vi "Dashboard Main.vi"() -> ()   [LabVIEW 2019]
uses:
  <vilib>/Rock Robotics/Network Tables/NT Read Numeric Array.vi
  <vilib>/Rock Robotics/Network Tables/NT Read String.vi
  max2018/dashboard/src/Robot Starting Location.ctl
panel:
  out "Camera Perf":string
  in  "Camera Settings":T1={"Frame Rate"=30, "Compression"=30, "Size"=1, "DB Camera Config"=FALSE} {"Frame Rate" scale=1.0..30.0; "Compression" scale=100.0..-1.0; "Size" items=["640x480", "320x240", "160x120"]}
  in  "TCP":refnum<k5>
  out "Robot IP":string
  in  "Dashboard Tab":enum32{"Drive", "Basic", "Custom", "Variables"}(tab)
  out "String":string
  in  "Robot Starting Location":enum32{"Left", "Centre", "Right", "Straight"}(radio)=enum."Centre"
  out "NT Connection":bool
  out "MotorChart R":cluster{"Numeric":dbl, "Numeric":dbl}(graph)
  out "MotorChart L":cluster{"Numeric":dbl, "Numeric":dbl}(graph)
  out "MotorSliders R":cluster{"MotorSlide1":dbl, "MotorSlide2":dbl} {"MotorSlide2" scale=-1.0..1.0 scale format="%#_2e"; "MotorSlide1" scale=-1.0..1.0 scale format="%#_2e"}
  out "MotorSliders L":cluster{"MotorSlide1":dbl, "MotorSlide2":dbl} {"MotorSlide2" scale=-1.0..1.0 scale format="%#_2e"; "MotorSlide1" scale=-1.0..1.0 scale format="%#_2e"}
  out "JS1 Z":dbl(slide) scale=-1.0..1.0 scale format="%#_2e"
  out "JS1 Graph":cluster{"X":dbl, "Y":dbl}[](graph)
  out "JS1 Buttons":T2
  out "JS2 Z":dbl(slide) scale=-1.0..1.0 scale format="%#_2e"
  out "JS2 Graph":cluster{"X":dbl, "Y":dbl}[](graph)
  out "JS2 Buttons":T2
  out "Mode":T3(ring)=enum."Auto Disabled"
  in  "DB/String 9":string
  in  "DB/String 8":string
  in  "DB/String 7":string
  in  "DB/String 6":string
  in  "DB/String 5":string
  in  "DB/String 4":string
  in  "DB/String 3":string
  in  "DB/String 2":string
  in  "DB/String 1":string
  in  "DB/String 0":string
  in  "DB/Slider 0":dbl(slide) scale=0.0..5.0
  in  "DB/Slider 1":dbl(slide) scale=0.0..5.0
  in  "DB/Slider 2":dbl(slide) scale=0.0..5.0
  in  "DB/Slider 3":dbl(slide) scale=0.0..5.0
  out "DB/LED 3":bool
  out "DB/LED 2":bool
  out "DB/LED 1":bool
  out "DB/LED 0":bool
  in  "DB/Button 3":bool
  in  "DB/Button 2":bool
  in  "DB/Button 1":bool
  in  "DB/Button 0":bool caption="New Name"
  out "Tree":string(tree)
  out "Camera Image":T4(plugin-control)
  in  "Camera Name":string(combo)="No Camera Selection"
  # "HW"
  # "Joysticks"
  # "Drive Motors"
  # "Front"
  # "Right"
  # "Left"
  # "Back"
  # "This tab is a great place for autonomous settings and robot-specific values.\nPlace controls and indicators inside this tab and match name to\nDashboard Variables on robot. You can also delete this comment."
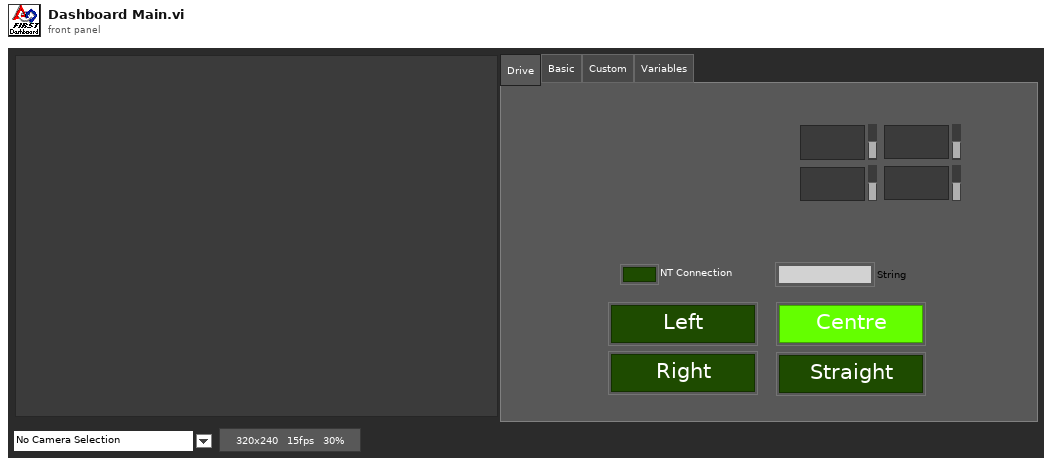
[diagram p1: front panel]
types:
  T1 = cluster{"Frame Rate":i32, "Compression":i32, "Size":u16, "DB Camera Config":bool}
  T2 = cluster{bool, bool, bool, bool, bool, bool, bool, bool, bool, bool, bool, bool}
  T3 = enum8{"Tele-Op Disabled", "Tele-Op Enabled", "Auto Disabled", "Auto Enabled", "Test Disabled", "Test Enabled", "Disconnected", "No Code", "E-Stop"}
  T4 = typedef "IMAQ Image.ctl" = refnum<image>
  T5 = typedef "Robot Starting Location.ctl" = enum32{"Left", "Centre", "Right"}
  T6 = cluster{"Save Path":path, "Interval (s)":dbl, "Keep":i32}
  T7 = typedef "Image Type" = u32
  T8 = cluster{"Camera Image":refnum<vi>, "Dashboard Tab":refnum<vi>, void, "Tree":refnum<vi>, "Camera Settings":refnum<vi>, "Camera Name":refnum<vi>, "Camera Perf":refnum<vi>}
  T9 = cluster{"Shift":bool, "Ctrl":bool, "Alt":bool, "Cmd":bool, "Opt":bool}
  T10 = cluster{"Error Strings":string, "Disable Counts":cluster{u16, u16}, "Rail Faults":cluster{u16, u16, u16}, "Robot IP":string, "DB Mode":u8, "Event Info":cluster{"Name":string, "Type":u8, "Number":u16, "Replay":u8}}
  T11 = cluster{"Storage":cluster{"Disk Free":u64, "RAM Block":u32, "RAM free":u32}, "CPU Utilization":cluster{"CPU % ISR":sgl, "CPU % Time Crit":sgl, "CPU % Timed Str":sgl, "CPU % High":sgl, "CPU % Above":sgl, "CPU % Normal":sgl, "CPU % Low":sgl}, "CAN":cluster{"% Bus Utilization":sgl, "Bus Off Cnt":u32, "TX_FIFO Full Cnt":u32, "Receive Error Cnt":u8, "Transmit Error Cnt":u8}, "HID":cluster{"HID Outputs":u32, "Rumble Low":u16, "Rumble High":u16}[]}
  T12 = cluster{"Status bits":cluster{"Test Mode":bool, "Autonomous":bool, "Enabled":bool, "Code Start":bool, "Brownout":bool, "Reserved 2":bool, "Reserved 3":bool, "E-Stop":bool}, "Code Trace":cluster{"Disabled":bool, "TeleOp":bool, "Auto":bool, "Test":bool}, "Controller Type":enum16{"unknown", "cRIO", "roboRio"}, "Code?":enum16{"unknown", "noCode", "code"}, "Battery V":dbl}
  T13 = cluster{"Control Bits":cluster{"TestMode":bool, "Autonomous":bool, "Enabled":bool, "FMS Present":bool, bool, bool, bool, "E-Stop":bool}, "Team Station ":u8, "Countdown":sgl, "Joystick Values":cluster{"Axes":dbl[], "Buttons":bool[], "POVs":i16[]}[]}
  T14 = cluster{"Axes":dbl[], "Buttons":bool[], "POVs":i16[]}[]
  T15 = cluster{"Axes":dbl[], "Buttons":bool[], "POVs":i16[]}
  T16 = cluster{"Buttons[0]":bool, "Buttons[1]":bool, "Buttons[2]":bool, "Buttons[3]":bool, "Buttons[4]":bool, "Buttons[5]":bool, "Buttons[6]":bool, "Buttons[7]":bool, "Buttons[8]":bool, "Buttons[9]":bool, "Buttons[10]":bool, "Buttons[11]":bool}
  T17 = cluster{"Camera Name":string, "Camera File Name":string, "Saved DB Images Info":cluster{"Save Path":path, "Interval (s)":dbl, "Keep":i32}}
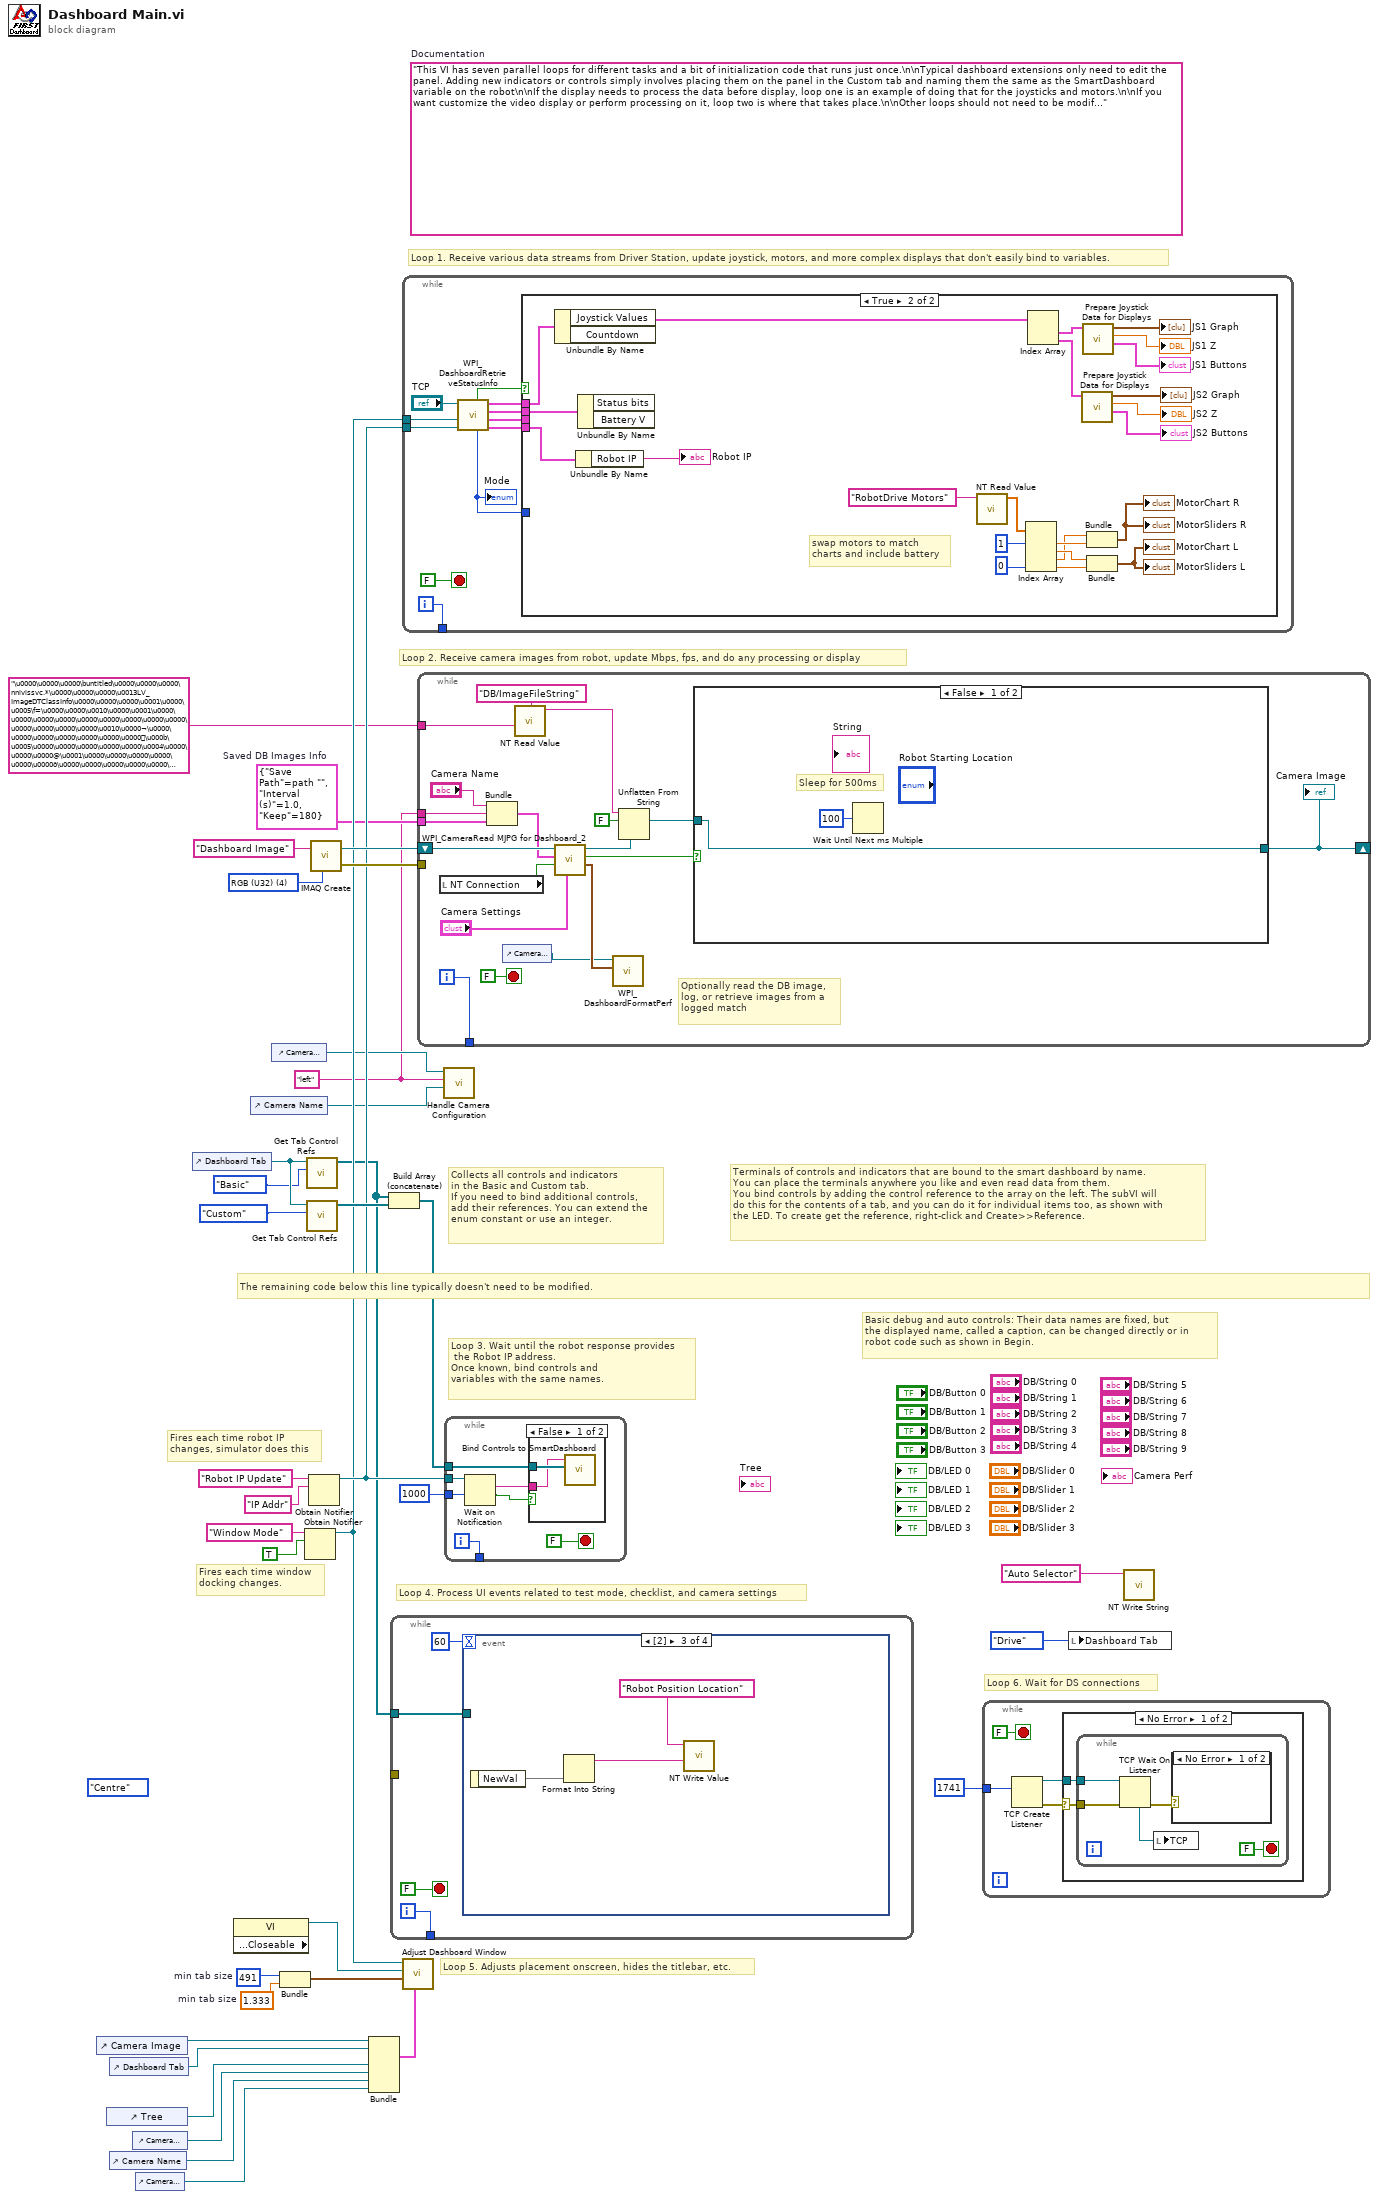
[diagram p0: block diagram]
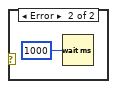
[diagram p2: hidden frame]
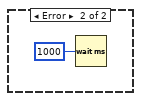
[diagram p3: hidden frame]
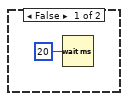
[diagram p4: hidden frame]
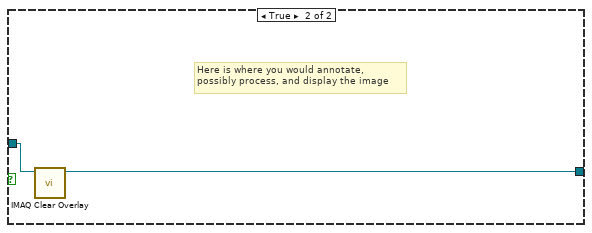
[diagram p6: hidden frame]
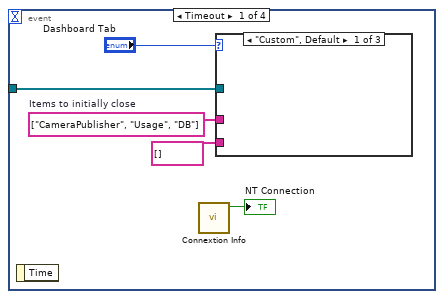
[diagram p7: hidden frame]
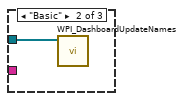
[diagram p8: hidden frame]
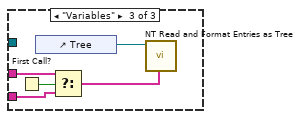
[diagram p9: hidden frame]
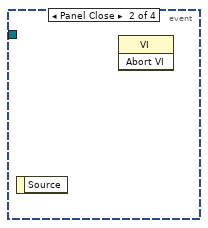
[diagram p10: hidden frame]
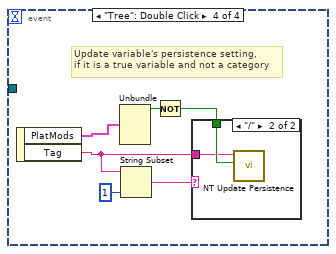
[diagram p11: hidden frame]
diagram:
  w2 = Robot_Starting_Location."Centre" ("Value (Signaling)")
  w4 = "left" ("Camera File Name")
  w5 = T6 {"Save Path"=path "", "Interval (s)"=1.0, "Keep"=180}  # Saved DB Images Info
  w25 = 491  # min tab size
  w24 = 1.333  # min tab size
  (unwired) "This VI has seven parallel loops for different tasks and a bit of initialization code that runs just once.\n\nTypical dashboard extensions only need to edit the panel. Adding new indicators or controls simply involves placing them on the panel in the Custom tab and naming them the same as the SmartDashboard variable on the robot\n\nIf the display needs to process the data before display, loop one is an example of doing that for the joysticks and motors.\n\nIf you want customize the video display or perform processing on it, loop two is where that takes place.\n\nOther loops should not need to be modified. They are pretty standard, and document the task they perform."  # Documentation
  w40 = T7 4 items=["Grayscale (U8)", "Grayscale (I16)", "Grayscale (SGL)", "Complex (CSG)", "RGB (U32)", "HSL (U32)", "RGB (U64)"] ("Image Type")
  # "Loop 6. Wait for DS connections"
  # "Basic debug and auto controls: Their data names are fixed, but\nthe displayed name, called a caption, can be changed directly or in\nrobot code such as shown in Begin."
  # "Fires each time robot IP\nchanges, simulator does this"
  # "Fires each time window\ndocking changes."
  # "Collects all controls and indicators\nin the Basic and Custom tab.\nIf you need to bind additional controls,\nadd their references. You can extend the\nenum constant or use an integer."
  # "The remaining code below this line typically doesn't need to be modified."
  # "Loop 4. Process UI events related to test mode, checklist, and camera settings"
  # "Terminals of controls and indicators that are bound to the smart dashboard by name.\nYou can place the terminals anywhere you like and even read data from them.\nYou bind controls by adding the control reference to the array on the left. The subVI will\ndo this for the contents of a tab, and you can do it for individual items too, as shown with\nthe LED. To create get the reference, right-click and Create>>Reference."
  # "Loop 3. Wait until the robot response provides\n the Robot IP address.\nOnce known, bind controls and\nvariables with the same names."
  # "Loop 5. Adjusts placement onscreen, hides the titlebar, etc."
  # "Loop 1. Receive various data streams from Driver Station, update joystick, motors, and more complex displays that don't easily bind to variables."
  # "Loop 2. Receive camera images from robot, update Mbps, fps, and do any processing or display"
  n1 = control-ref of="Camera Image"() -> (w27:refnum<vi>)
  n2 = control-ref of="Tree"() -> (w11:refnum<vi>)
  n3 = control-ref of="Dashboard Tab"() -> (w26:refnum<vi>)
  n4 = control-ref of="Camera Name"() -> (w9:refnum<vi>)
  n5 = control-ref of="Camera Settings"() -> (w10:refnum<vi>)
  n6 = control-ref of="Camera Perf"() -> (w8:refnum<vi>)
  n7 = control-ref of="Dashboard Tab"() -> (w30:refnum<vi>)
  n8 = property class="VI" props=["Front Panel.Closeable"]() -> (reference out=w31:refnum<vi>)  [unwired: 2 in, 2 out]
  n9 = control-ref of="Camera Name"() -> (w15:refnum<vi>)
  n10 = control-ref of="Camera Settings"() -> (w16:refnum<vi>)
  n11 = Bundle("min tab size"=w25, "min tab size"=w24) -> (w23:cluster{"min tab size":i32, "min tab size":dbl})  [unwired: 1 in]
  n12 = Obtain Notifier(name (unnamed)="Window Mode", notification data type=TRUE) -> (notifier out=w19:refnum<notifier>)  [unwired: 2 in, 2 out]
  n13 = call <vilib>:"Get Tab Control Refs.vi"("Page Index"=enum32{"Drive", "Basic", "Custom", "Variables"}."Basic" ("Dashboard Tab"), "TabControl in"=w30) -> ("ControlsOnPage"=w14:refnum<vi>[])  [unwired: 9 in]
  n14 = call <vilib>:"Get Tab Control Refs.vi"("Page Index"=enum32{"Drive", "Basic", "Custom", "Variables"}."Custom" ("Dashboard Tab"), "TabControl in"=w30) -> ("ControlsOnPage"=w29:refnum<vi>[])  [unwired: 9 in]
  n15 = Obtain Notifier(name (unnamed)="Robot IP Update", notification data type="IP Addr" ("name (unnamed)")) -> (notifier out=w20:refnum<notifier>)  [unwired: 2 in, 2 out]
  n16 = call "IMAQ Create"("Image Name"="Dashboard Image", "Image Type"=w40) -> ("New Image"=w38:T4, "error out"=w37:errorcluster)  [unwired: 2 in, 1 out]
  n17 = Bundle("Camera Image"=w27, "Dashboard Tab"=w26, "Tree"=w11, "Camera Settings"=w10, "Camera Name"=w9, "Camera Perf"=w8) -> (w21:T8, w22)  [unwired: 1 in]
  n18 = Build Array (concatenate)(w14, w29) -> (w28:refnum<vi>[])
  n19 = while {
    tunnel: [w42] -> _
    tunnel: w14 -> [w41]
    tunnel: [_] -> w1
    i -> [w42]
    stop <- FALSE stop-if-true
    n20 = event shown="[2]" {
      selector: _ -> [_ _ _ _]
      dyn-events: _ -> [_ _ _ _]
      timeout: u32 60 ("milliseconds to wait") -> [_ _ _ _]
      tunnel: w41 -> [w47 _ _ _]
      event Timeout {
        w46 = string[] ["CameraPublisher", "Usage", "DB"]  # Items to initially close
        n21 = event-data() -> ()  [unwired: 1 in, 1 out]
        n22 = call <vilib>:"Connextion Info.vi"() -> ("Connected"=→"NT Connection":bool)  [unwired: 10 in, 1 out]
        n23 = case shown="\"Custom\", Default" "Dashboard Tab" {
          tunnel: w47 -> [_ w50 _]
          tunnel: w46 -> [_ _ w53]
          tunnel: string[] [] -> [_ _ w52]
          frame "Custom", Default {
          }
          frame "Basic" {
            n24 = call <vilib>:"WPI_DashboardUpdateNames.vi"("Controls on Tab"=w50) -> ()  [unwired: 11 in]
          }
          frame "Variables" {
            n25 = First Call?() -> (First Call?: T/F=w54:bool)
            n26 = control-ref of="Tree"() -> (w55:refnum<vi>)
            n27 = Select(t=w53, s=w54, f=w52) -> (s? t:f=w51:string[])
            n28 = call <vilib>:"NT Read and Format Entries as Tree.vi"("Tags to  Close"=w51, "Tree Refnum"=w55) -> ()  [unwired: 8 in, 2 out]
          }
        }
      }
      event Panel Close {
        n29 = event-data() -> ()  [unwired: 1 in, 1 out]
        n30 = invoke class="VI" method="Abort VI"() -> ()  [unwired: 3 in, 3 out]
      }
      event #2 (no event record) {
        n31 = event-data() -> ("NewVal"=w58)  [unwired: 1 in]
        n32 = Format Into String(w58) -> (resulting string=w56:string)  [unwired: 3 in, 1 out]
        n33 = call-poly <vilib>:"NT Write Value.vi"("String"=w56, "Name"="Robot Position Location") -> ()  [unwired: 9 in, 1 out]
      }
      event "Tree": Double Click {
        # "Update variable's persistence setting,\nif it is a true variable and not a category"
        n34 = event-data() -> ("PlatMods"=w60:T9, "Tag"=w59:string)  [unwired: 1 in]
        n35 = Unbundle(w60) -> ("Shift"=w64:bool)  [unwired: 4 out]
        n36 = String Subset(string=w59, length (rest)=1 ("length (rest)")) -> (substring=w61:string)  [unwired: 1 in]
        n37 = Not(x=w64) -> (.not. x?=w63:bool)
        n38 = case shown="\"/\"" w61 {
          tunnel: w63 -> [_ w66]
          tunnel: w59 -> [_ w65]
          frame Default {
          }
          frame "/" {
            n39 = call <vilib>:"NT Update Persistence.vi"("Persistence"=w66, "Name"=w65) -> ()  [unwired: 9 in, 1 out]
          }
        }
      }
    }
  }
  n40 = while {
    tunnel: [w76] -> _
    tunnel: w20 -> [w70]
    tunnel: w19 -> [w67]
    i -> [w76]
    stop <- FALSE stop-if-true
    n41 = call <vilib>:"WPI_DashboardRetrieveStatusInfo.vi"("Binding Refnum"=w70, "Window Mode Notifier"=w67, "TCP Cnx"="TCP") -> ("Power and Errors"=w71:T10, "Robot Metrics"=w74:T11, "Status Info"=w75:T12, "Control Info"=w72:T13, "Robot Mode"=w69:T3, "Process?"=w73:bool)  [unwired: 3 in]
    "Mode" <- w69
    n42 = case shown="True" w73 {
      tunnel: w75 -> [_ w101]
      tunnel: w74 -> [_ _]
      tunnel: w72 -> [_ w100]
      tunnel: w71 -> [_ w99]
      tunnel: w69 -> [_ _]
      frame False {
        n43 = Wait (ms)(milliseconds to wait=u32 20) -> ()  [unwired: 1 out]
      }
      frame True {
        # "swap motors to match\ncharts and include battery"
        n44 = Unbundle By Name(w100) -> ("Joystick Values"=w90:T14)  [unwired: 1 out]
        n45 = Unbundle By Name(w99) -> ("Robot IP"=→"Robot IP":string)
        n46 = Unbundle By Name(w101) -> ()  [unwired: 2 out]
        n47 = call-poly <vilib>:"NT Read Value.vi"("Name"="RobotDrive Motors") -> ("Numeric Array"=w80:dbl[])  [unwired: 9 in, 1 out]
        n48 = Index Array(array=w80, index #1=1, index #4=0) -> (element #1=w94:dbl, element #2=w95:dbl, element #3=w93:dbl, element #4=w98:dbl)  [unwired: 2 in]
        n49 = Index Array(array=w90) -> (element #1=w89:T15, element #2=w85:T15)  [unwired: 2 in]
        n50 = call "Prepare Joystick Data for Displays.vi"("Joystick Values"=w85) -> ("Buttons"=→"JS2 Buttons":T16, "Z Axis"=→"JS2 Z":dbl, "Cartesian Data"=→"JS2 Graph":cluster{"X axis":dbl, "X axis":dbl}[])  [unwired: 8 in]
        n51 = call "Prepare Joystick Data for Displays.vi"("Joystick Values"=w89) -> ("Buttons"=→"JS1 Buttons":T16, "Z Axis"=→"JS1 Z":dbl, "Cartesian Data"=→"JS1 Graph":cluster{"X axis":dbl, "X axis":dbl}[])  [unwired: 8 in]
        n52 = Bundle("Numeric"=w93, "Numeric"=w94) -> (→"MotorChart R" →"MotorSliders R":cluster{"Numeric":dbl, "Numeric":dbl})  [unwired: 1 in]
        n53 = Bundle("Numeric"=w95, "Numeric"=w98) -> (→"MotorChart L" →"MotorSliders L":cluster{"Numeric":dbl, "Numeric":dbl})  [unwired: 1 in]
      }
    }
  }
  n54 = call "Adjust Dashboard Window.vi"("Sizing Refnums"=w21, "Size Constraints"=w23, "VI"=w31, "WIn Mode"=w19) -> ()  [unwired: 8 in]
  n55 = while {
    tunnel: w37 -> [_]
    tunnel: [w119] -> _
    tunnel: w5 -> [w114]
    tunnel: w4 -> [w111]
    tunnel: "\u0000\u0000\u0000\buntitled\u0000\u0000\u0000\nnivissvc.*\u0000\u0000\u0000\u0013LV_ImageDTClassInfo\u0000\u0000\u0000\u0001\u0000\u0005\f=\u0000\u0000\u0010\u0000\u0001\u0000\u0000\u0000\u0000\u0000\u0000\u0000\u0000\u0000\u0000\u0000\u0000\u0000\u0010\u0000¬\u0000\u0000\u0000\u0000\u0000\u0000\u0000\u000b\u0005\u0000\u0000\u0000\u0000\u0000\u0004\u0000\u0000\u0000@\u0001\u0000\u0000\u0000\u0000\u0000\u0000ð\u0000\u0000\u0000\u0000\u0000\u0000\u0000\u0003\u0000\u0000\u0000\u0000\u0000\u0000\u0000\u0000\u0000\u0000\u0000\u0000\u0000\u0000\u0000\u0000\u0000\u0000\u0000\u0000\u0000\u0000\u0000\u0000\u0000\u0000\u0000P\u0001\u0000\u0000\u0000\u0000\u0000\u0000\u0000\u0000\u0000\u0000ø\bg\u0013\u0000\u0000\u0000\u0000¤¾\u0019\u0000\u0000\u0000\u0000@l@O\u0000\u0000°\u0012\u0000\u0000\u0000\u0000\u0000\u0000\u0000\u0000\u0000\u0000\u0001\u0000\u0000\u0000\u0001\u0000\u0000\u0000\u0000\u0000\u0000\u0000\b\u0000\u0000\u0000\u000b\u0005\u0000\u0000\u0000\u0000\u0000\u0000\u0000\u0000\u0000\u0000\u0000\u0000\u0000\t\u0000\u0000\u0000\u0000\u0000\u0000\u0000untitled\u0000\u0000\u0000\u0000\u0000\u0000\u0000\u0000\u0000\u0000\u0000\u0000\u0000\u0000\u0000\u0000\u0000\u0000\u0000\u0000\u0000\u0000\u0000\u0000\u0000\u0000\u0000\u0000\u0000\u0000\u0000\u0000\u0000\u0000\u0000\u0000\u0000\u0000\u0000\u0000\u0000\u0000\u0000\u0000\u0000\u0000\u0000\u0000\u0000\u0000\u0000\u0000\u0000\u0000\u0000\u0000\u0000\u0000\u0000\u0000\u0000\u0000\u0000\u0000\u0000\u0000\u0000\u0000\u0000\u0000\u0000\u0000\u0000\u0000\u0000\u0000\u0000\u0000\u0000\u0000\u0000\u0000\u0000\u0000\u0000\u0000\u0000\u0000\u0000\u0000\u0000\u0000\u0000\u0000\u0000\u0000\u0000\u0000\u0000\u0000\u0000\u0000\u0000\u0000\u0000\u0000\u0000\u0000\u0000\u0000\u0000\u0000\u0000\u0000\u0000\u0000\u0000\u0000\u0000\u0000\u0000\u0000\u0000\u0000\u0000\u0000\u0000\u0000\u0000\u0000\u0000\u0000\u0000\u0000\u0000\u0000\u0000\u0000\u0000\u0000\u0000\u0000\u0000\u0000\u0000\u0000\u0000\u0000\u0000\u0000\u0000\u0000\u0000\u0000\u0000\u0000\u0000\u0000\u0000\u0000\u0000\u0000\u0000\u0000\u0000\u0000\u0000\u0000\u0000\u0000\u0000\u0000\u0000\u0000\u0000\u0000\u0000\u0000\u0000\u0000\u0000\u0000\u0000\u0000\u0000\u0000\u0000\u0000\u0000\u0000\u0000\u0000\u0000\u0000\u0000\u0000\u0000\u0000\u0000\u0000\u0000\u0000\u0000\u0000\u0000\u0000\u0000\u0000\u0000\u0000\u0000\u0000\u0000\u0000\u0000\u0000\u0000\u0000\u0000\u0000\u0000\u0000\u0000\u0000\u0000\u0000\u0000\u0000\u0000\u0000\u0000\u0000\u0000\u0000\u0000\u0000\u0000\u0000\u0000\u0000\u0000\u0000\u0000\u0000\u0000\u0000\u0000\u0000\u0000\u0000\u0000\u0000\u0000\u0000\u0000\u0000\u0000\u0000\u0000\u0000\u0000\u0000\u0000\u0000\u0000\u0000\u0000\u0000\u0000\u0000\u0000\u0000\u0000\u0000\u0000\u0000\u0000\u0000\u0000\u0000\u0000\u0000\u0000\u0000\u0000\u0000\u0000\u0000\u0000\u0000\u0000\u0000\u0000\u0000\u0000\u0000\u0000\u0000\u0000\u0000\u0000\u0000\u0000\u0000\u0000\u0000\u0000\u0000\u0000\u0000\u0000\u0000\u0000\u0000\u0000\u0000\u0000\u0000\u0000\u0000\u0000\u0000\u0000\u0000\u0000\u0000\u0000\u0000\u0000\u0000\u0000\u0000\u0000\u0000\u0000\u0000\u0000\u0000\u0000\u0000\u0000\u0000\u0000\u0000\u0000\u0000\u0000\u0000\u0000\u0000\u0000\u0000\u0000\u0000\u0000\u0000\u0000\u0000\u0000\u0000\u0000\u0000\u0000..." ("Data String") -> [w105]
    shift-right: [w102] -> _
    shift-left: w38 -> [w118]
    i -> [w119]
    stop <- FALSE stop-if-true
    # "Optionally read the DB image,\nlog, or retrieve images from a\nlogged match"
    n56 = local read "NT Connection"() -> (w115:bool)
    n57 = Bundle("Camera Name"="Camera Name", "Camera File Name"=w111, "Saved DB Images Info"=w114) -> (w113:T17)  [unwired: 1 in]
    n58 = control-ref of="Camera Perf"() -> (w109:refnum<vi>)
    n59 = call-poly <vilib>:"NT Read Value.vi"("Default Value"=w105, "Name"="DB/ImageFileString") -> ("String"=w104:string)  [unwired: 8 in, 1 out]
    n60 = call <vilib>:"WPI_CameraRead MJPG for Dashboard_2.vi"("Camera Settings"="Camera Settings", "NT Connection"=w115, "Capture Info"=w113, "Image in"=w118) -> ("perf info"=w110:cluster{"Bandwidth (Mbps)":dbl, "fps":dbl}, "Active"=w117:bool, "Image\\ out"=w108:T4)  [unwired: 5 in]
    n61 = call <vilib>:"WPI_DashboardFormatPerf.vi"("Performance"=w110, "String in"=w109) -> ()  [unwired: 10 in]
    n62 = Unflatten From String(type=w108, binary string=w104, data includes array or string size? (T)=FALSE) -> (value=w103:T4)  [unwired: 2 in, 2 out]
    n63 = case shown="False" w117 {
      tunnel: [w121 w124] -> w102
      tunnel: w103 -> [w121 w123]
      frame False {
        # "Sleep for 500ms"
        n64 = Wait Until Next ms Multiple(millisecond multiple=u32 100) -> ()  [unwired: 1 out]
      }
      frame True {
        # "Here is where you would annotate,\npossibly process, and display the image"
        n65 = call "IMAQ Clear Overlay"("Image"=w123) -> ("Image Out"=w124:T4)  [unwired: 2 in, 8 out]
      }
    }
    "Camera Image" <- w102
  }
  n66 = call "Handle Camera Configuration.vi"("CameraNameRef"=w15, "Display Name"=w4, "ClusterRef"=w16) -> ()  [unwired: 9 in]
  n67 = while {
    tunnel: w28 -> [w131]
    tunnel: w20 -> [w129]
    tunnel: [w127] -> _
    tunnel: u32 1000 ("milliseconds to wait") -> [w126]
    i -> [w127]
    stop <- FALSE stop-if-true
    n68 = Wait on Notification(notifier=w129, timeout in ms (-1)=w126) -> (notification=w128:string, timed out?=w125:bool)  [unwired: 2 in, 2 out]
    n69 = case shown="False" w125 {
      tunnel: w131 -> [w133 _]
      tunnel: w128 -> [w132 _]
      frame False {
        n70 = call <vilib>:"Bind Controls to SmartDashboard.vi"("Bound Control Refs"=w133, "Server IP Address"=w132) -> ()  [unwired: 10 in]
      }
      frame True {
      }
    }
  }
  n71 = while {
    tunnel: u16 1741 ("timeout ms (25000)") -> [w135]
    stop <- FALSE stop-if-true
    n72 = TCP Create Listener(10:w135) -> (0:w134:errorcluster, 3:w136:refnum<k5>)  [unwired: 4 in, 1 out]
    n73 = case shown="No Error" w134 {
      selector: w134 -> [w138 _]
      tunnel: w136 -> [w139 _]
      frame No Error {
        n74 = while {
          tunnel: w139 -> [w142]
          tunnel: w138 -> [w141]
          stop <- FALSE stop-if-true
          n75 = TCP Wait On Listener(8:w141, 11:w142) -> (0:w143:errorcluster, 4:w144:refnum<k5>)  [unwired: 2 in, 3 out]
          n76 = local write "TCP"(w144) -> ()
          n77 = case shown="No Error" w143 {
            frame No Error {
            }
            frame Error {
              n78 = Wait (ms)(milliseconds to wait=u32 1000) -> ()  [unwired: 1 out]
            }
          }
        }
      }
      frame Error {
        n79 = Wait (ms)(milliseconds to wait=u32 1000) -> ()  [unwired: 1 out]
      }
    }
  }
  n80 = local write "Dashboard Tab"(enum32{"Drive", "Basic", "Custom", "Variables"}."Drive" ("Dashboard Tab")) -> ()
  n81 = call <vilib>:"NT Write String.vi"("Name"="Auto Selector") -> ("String"=w12:string)  [unwired: 9 in, 1 out]
